vi "XYMEAN(SubVI).vi"(1 "Object Size":u32, 2 "Position Analysis Report":cluster{"x":sgl, "y":sgl} {"y" format="%.2f"; "x" format="%.2f"}, 3 "Position Match Shape":cluster{"x":sgl, "y":sgl} {"y" format="%.2f"; "x" format="%.2f"}, 4 "Position Match Color":cluster{"x":sgl, "y":sgl} {"y" format="%.2f"; "x" format="%.2f"}) -> (0 "Result":T1 {"Variance"."Ey2" format="%.2f"; "Variance"."Ex2" format="%.2f"; "Standar Desviation"."Ey" format="%.2f"; "Standar Desviation"."Ex" format="%.2f"; "Position"."Y" format="%.2f"; "Position"."X" format="%.2f"})   [LabVIEW 2011]
doc: "Calcula la media con error de tres posiciones."
uses:
  NI_AALBase.lvlib
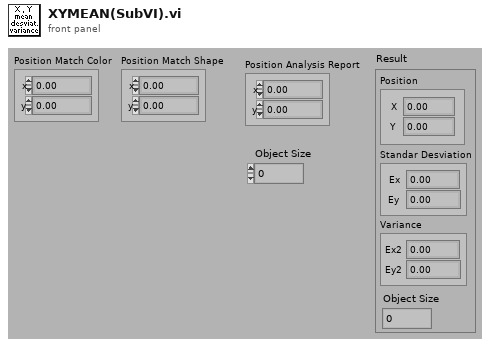
[diagram p1: front panel]
types:
  T1 = cluster{"Position":cluster{"X":sgl, "Y":sgl}, "Standar Desviation":cluster{"Ex":sgl, "Ey":sgl}, "Variance":cluster{"Ex2":sgl, "Ey2":sgl}, "Object Size":u32}
  T2 = cluster{cluster{"mean":dbl, "mean":dbl}, cluster{"mean":dbl, "mean":dbl}, cluster{"mean":dbl, "mean":dbl}, "Object Size":u32}
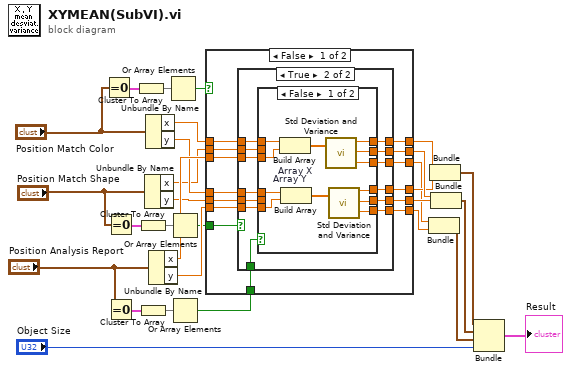
[diagram p0: block diagram]
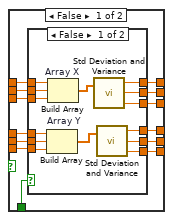
[diagram p2: hidden frame]
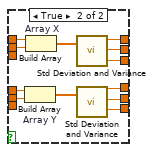
[diagram p3: hidden frame]
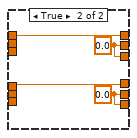
[diagram p4: hidden frame]
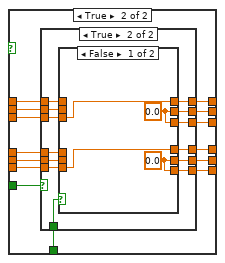
[diagram p5: hidden frame]
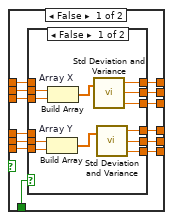
[diagram p6: hidden frame]
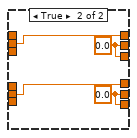
[diagram p7: hidden frame]
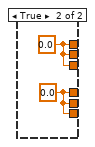
[diagram p8: hidden frame]
diagram:
  n1 = Equal To 0?(x="Position Match Color") -> (x = 0?=w15:cluster{"x":bool, "y":bool})
  n2 = Equal To 0?(x="Position Match Shape") -> (x = 0?=w18:cluster{"x":bool, "y":bool})
  n3 = Equal To 0?(x="Position Analysis Report") -> (x = 0?=w21:cluster{"x":bool, "y":bool})
  n4 = Cluster To Array(cluster=w15) -> (array=w16:bool[])
  n5 = Cluster To Array(cluster=w18) -> (array=w19:bool[])
  n6 = Cluster To Array(cluster=w21) -> (array=w22:bool[])
  n7 = Unbundle By Name("Position Match Shape") -> ("x"=w10:sgl, "y"=w9:sgl)
  n8 = Unbundle By Name("Position Match Color") -> ("x"=w13:sgl, "y"=w14:sgl)
  n9 = Unbundle By Name("Position Analysis Report") -> ("x"=w23:sgl, "y"=w24:sgl)
  n10 = Or Array Elements(Boolean array=w16) -> (logical OR=w17:bool)
  n11 = Or Array Elements(Boolean array=w19) -> (logical OR=w20:bool)
  n12 = Or Array Elements(Boolean array=w22) -> (logical OR=w27:bool)
  n13 = case shown="False" w17 {
    tunnel: w9 -> [w43 w122]
    tunnel: w10 -> [w42 w119]
    tunnel: [w41 w115] -> w11
    tunnel: [w40 w112] -> w12
    tunnel: w13 -> [w39 w118]
    tunnel: w14 -> [w38 w121]
    tunnel: w20 -> [w37 w125]
    tunnel: w23 -> [w36 w120]
    tunnel: w24 -> [w35 w123]
    tunnel: [w34 w113] -> w25
    tunnel: [w33 w116] -> w26
    tunnel: w27 -> [w32 w124]
    tunnel: [w31 w114] -> w3
    tunnel: [w30 w117] -> w2
    frame False {
      n14 = case shown="True" w37 {
        tunnel: w43 -> [w56 w91]
        tunnel: w42 -> [w55 w94]
        tunnel: [w54 w86] -> w41
        tunnel: [w53 w83] -> w40
        tunnel: w39 -> [w52 w95]
        tunnel: w38 -> [w51 w92]
        tunnel: w36 -> [w50 w93]
        tunnel: w35 -> [w49 w90]
        tunnel: [w48 w84] -> w34
        tunnel: [w47 w87] -> w33
        tunnel: w32 -> [w46 w89]
        tunnel: [w45 w85] -> w31
        tunnel: [w44 w88] -> w30
        frame False {
          n15 = case shown="False" w46 {
            tunnel: w56 -> [w70 w75]
            tunnel: w55 -> [w69 w77]
            tunnel: [w68 w79] -> w54
            tunnel: [w67 w80] -> w53
            tunnel: w52 -> [w66 w78]
            tunnel: w51 -> [w65 w76]
            tunnel: w50 -> [w62 _]
            tunnel: w49 -> [w61 _]
            tunnel: [w60 w74] -> w48
            tunnel: [w59 w72] -> w47
            tunnel: [w58 w73] -> w45
            tunnel: [w57 w71] -> w44
            frame False {
              n16 = Build Array "Array Y"(w65, w70, w61) -> (w63:sgl[])
              n17 = Build Array "Array X"(w66, w69, w62) -> (w64:sgl[])
              n18 = call "Std Deviation and Variance.vi"("X"=w64) -> ("mean"=w67:dbl, "standard deviation"=w60:dbl, "variance"=w58:dbl)  [unwired: 1 in]
              n19 = call "Std Deviation and Variance.vi"("X"=w63) -> ("mean"=w68:dbl, "standard deviation"=w59:dbl, "variance"=w57:dbl)  [unwired: 1 in]
            }
            frame True {
              n20 = Build Array "Array Y"(w76, w75) -> (w81:sgl[])
              n21 = Build Array "Array X"(w78, w77) -> (w82:sgl[])
              n22 = call "Std Deviation and Variance.vi"("X"=w82) -> ("mean"=w80:dbl, "standard deviation"=w74:dbl, "variance"=w73:dbl)  [unwired: 1 in]
              n23 = call "Std Deviation and Variance.vi"("X"=w81) -> ("mean"=w79:dbl, "standard deviation"=w72:dbl, "variance"=w71:dbl)  [unwired: 1 in]
            }
          }
        }
        frame True {
          n24 = case shown="False" w89 {
            tunnel: w91 -> [_ _]
            tunnel: w94 -> [_ _]
            tunnel: [w104 w108] -> w86
            tunnel: [w105 w109] -> w83
            tunnel: w95 -> [w98 w109]
            tunnel: w92 -> [w96 w108]
            tunnel: w93 -> [w97 _]
            tunnel: w90 -> [w99 _]
            tunnel: [w103 w111] -> w84
            tunnel: [w101 w110] -> w87
            tunnel: [w102 w111] -> w85
            tunnel: [w100 w110] -> w88
            frame False {
              n25 = Build Array "Array X"(w98, w97) -> (w107:sgl[])
              n26 = Build Array "Array Y"(w96, w99) -> (w106:sgl[])
              n27 = call "Std Deviation and Variance.vi"("X"=w107) -> ("mean"=w105:dbl, "standard deviation"=w103:dbl, "variance"=w102:dbl)  [unwired: 1 in]
              n28 = call "Std Deviation and Variance.vi"("X"=w106) -> ("mean"=w104:dbl, "standard deviation"=w101:dbl, "variance"=w100:dbl)  [unwired: 1 in]
            }
            frame True {
              w110 = 0.0 ("standard deviation")
              w111 = 0.0 ("standard deviation")
            }
          }
        }
      }
    }
    frame True {
      n29 = case shown="True" w125 {
        tunnel: w122 -> [w138 w162]
        tunnel: w119 -> [w137 w165]
        tunnel: [w136 w157] -> w115
        tunnel: [w135 w160] -> w112
        tunnel: w118 -> [w134 w166]
        tunnel: w121 -> [w133 w163]
        tunnel: w120 -> [w132 w164]
        tunnel: w123 -> [w131 w161]
        tunnel: [w130 w159] -> w113
        tunnel: [w129 w156] -> w116
        tunnel: w124 -> [w128 w167]
        tunnel: [w127 w158] -> w114
        tunnel: [w126 w155] -> w117
        frame False {
          n30 = case shown="False" w128 {
            tunnel: w138 -> [w150 w153]
            tunnel: w137 -> [w149 w154]
            tunnel: [w148 w153] -> w136
            tunnel: [w147 w154] -> w135
            tunnel: w134 -> [_ _]
            tunnel: w133 -> [_ _]
            tunnel: w132 -> [w144 _]
            tunnel: w131 -> [w143 _]
            tunnel: [w142 w151] -> w130
            tunnel: [w141 w152] -> w129
            tunnel: [w140 w151] -> w127
            tunnel: [w139 w152] -> w126
            frame False {
              n31 = Build Array "Array Y"(w150, w143) -> (w145:sgl[])
              n32 = Build Array "Array X"(w149, w144) -> (w146:sgl[])
              n33 = call "Std Deviation and Variance.vi"("X"=w146) -> ("mean"=w147:dbl, "standard deviation"=w142:dbl, "variance"=w140:dbl)  [unwired: 1 in]
              n34 = call "Std Deviation and Variance.vi"("X"=w145) -> ("mean"=w148:dbl, "standard deviation"=w141:dbl, "variance"=w139:dbl)  [unwired: 1 in]
            }
            frame True {
              w151 = 0.0 ("standard deviation")
              w152 = 0.0 ("standard deviation")
            }
          }
        }
        frame True {
          n35 = case shown="False" w167 {
            tunnel: w162 -> [_ _]
            tunnel: w165 -> [_ _]
            tunnel: [w171 w172] -> w157
            tunnel: [w170 w173] -> w160
            tunnel: w166 -> [_ _]
            tunnel: w163 -> [_ _]
            tunnel: [w169 w173] -> w159
            tunnel: [w168 w172] -> w156
            tunnel: [w169 w173] -> w158
            tunnel: [w168 w172] -> w155
            tunnel: w164 -> [w170 _]
            tunnel: w161 -> [w171 _]
            frame False {
              w168 = 0.0 ("mean")
              w169 = 0.0 ("mean")
            }
            frame True {
              w172 = 0.0 ("mean")
              w173 = 0.0 ("mean")
            }
          }
        }
      }
    }
  }
  n36 = Bundle("mean"=w3, "mean"=w2) -> (w4:cluster{"mean":dbl, "mean":dbl})  [unwired: 1 out]
  n37 = Bundle("mean"=w12, "mean"=w11) -> (w28:cluster{"mean":dbl, "mean":dbl})  [unwired: 1 out]
  n38 = Bundle("mean"=w25, "mean"=w26) -> (w29:cluster{"mean":dbl, "mean":dbl})  [unwired: 1 out]
  n39 = Bundle(w28, w29, w4, "Object Size"="Object Size") -> (→"Result":T2)  [unwired: 1 out]
